vi "AmplitudeModulation.vi"() -> ()   [LabVIEW 2015]
uses:
  <vilib>/DAQmx/read.llb/DAQmx Read (Analog 1D DBL NChan 1Samp).vi
  <vilib>/DAQmx/miscellaneous.llb/DAQmx Fill In Error Info.vi
  <vilib>/addons/control/pid/pid.llb/PID (DBL).vi
  <instrlib>/Agilent 33XXX Series/Agilent 33XXX Series.lvlib
  <vilib>/addons/control/pid/NI_PID_pid.lvlib
  <vilib>/ptbypt/NI_PtbyPt.lvlib
panel:
  in  "View Saved Data\nUpon Completion":bool=TRUE
  out "Time Elapsed (s)":u32
  out "Temperature":dbl[](graph) caption="Signals"
  in  "Slide":dbl(slide) scale=35.0..45.0
  in  "Start":bool
  out "Actual Samp\nRate (Hz)":dbl format="%#_2g"
  in  "Feed back Mechanism":enum32{"PID Control", "Simple P Control"}(tab)
  in  "PID gains":T1={"proportional gain (Kc)"=0.03, "integral time (Ti, min)"=0.175, "derivative time (Td, min)"=0.003} {"derivative time (Td, min)" format="%.3f"; "integral time (Ti, min)" format="%.3f"; "proportional gain (Kc)" format="%.3f"}
  in  "Simple P":dbl
  in  "Amplitude\nModulation?":bool=TRUE
  in  "voltage limit":dbl=0.3 format="%#_13g"
  in  "Set Point (C)":dbl=40.0
  in  "Total Time (s)":u32=300
  in  "Output":bool=TRUE
  in  "Amplitude (V)":dbl=0.2 format="%#_3g"
  in  "Stop":bool
  out "Current Reading":dbl=34.489131869267396 format="%#.1g"
  out "Waveform Chart":waveform(dbl)(graph)
  in  "Log Data?":bool=TRUE
  in  "Description":string="Test Data. See Pictures."
  in  "File Path":path=path "C:/Data/Sonify Labview/ChickenWithChillerWithStandoff.lvm" caption="Filename"
  # "(Set Point - Current Reading) * P\n+ Current Voltage\n= New Voltage"
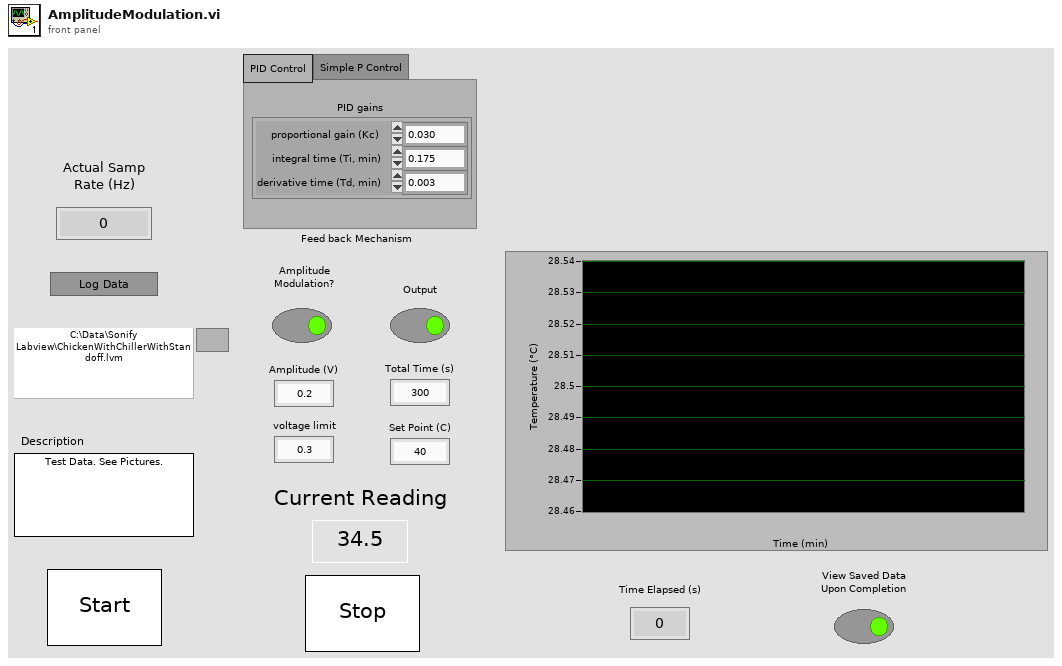
[diagram p1: front panel]
types:
  T1 = cluster{"proportional gain (Kc)":dbl, "integral time (Ti, min)":dbl, "derivative time (Td, min)":dbl}
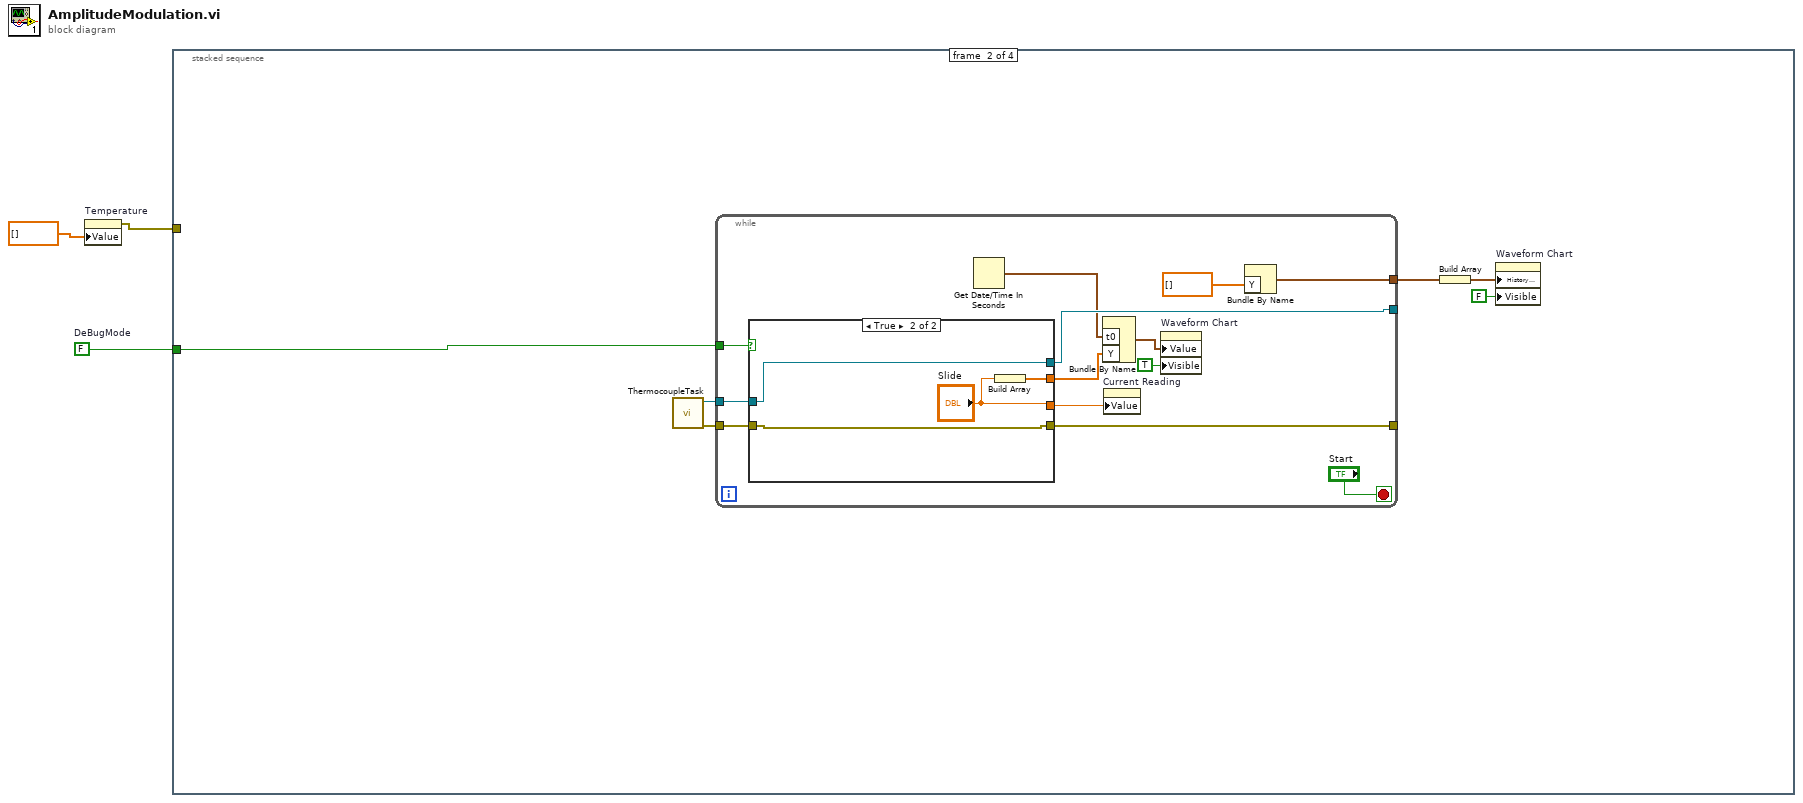
[diagram p0: block diagram]
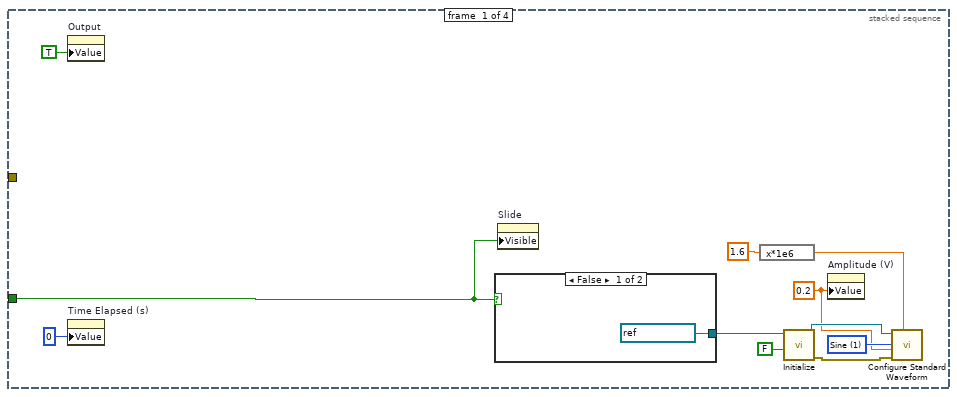
[diagram p2: hidden frame]
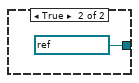
[diagram p3: hidden frame]
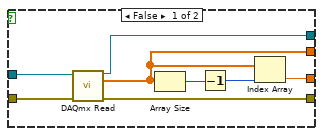
[diagram p4: hidden frame]
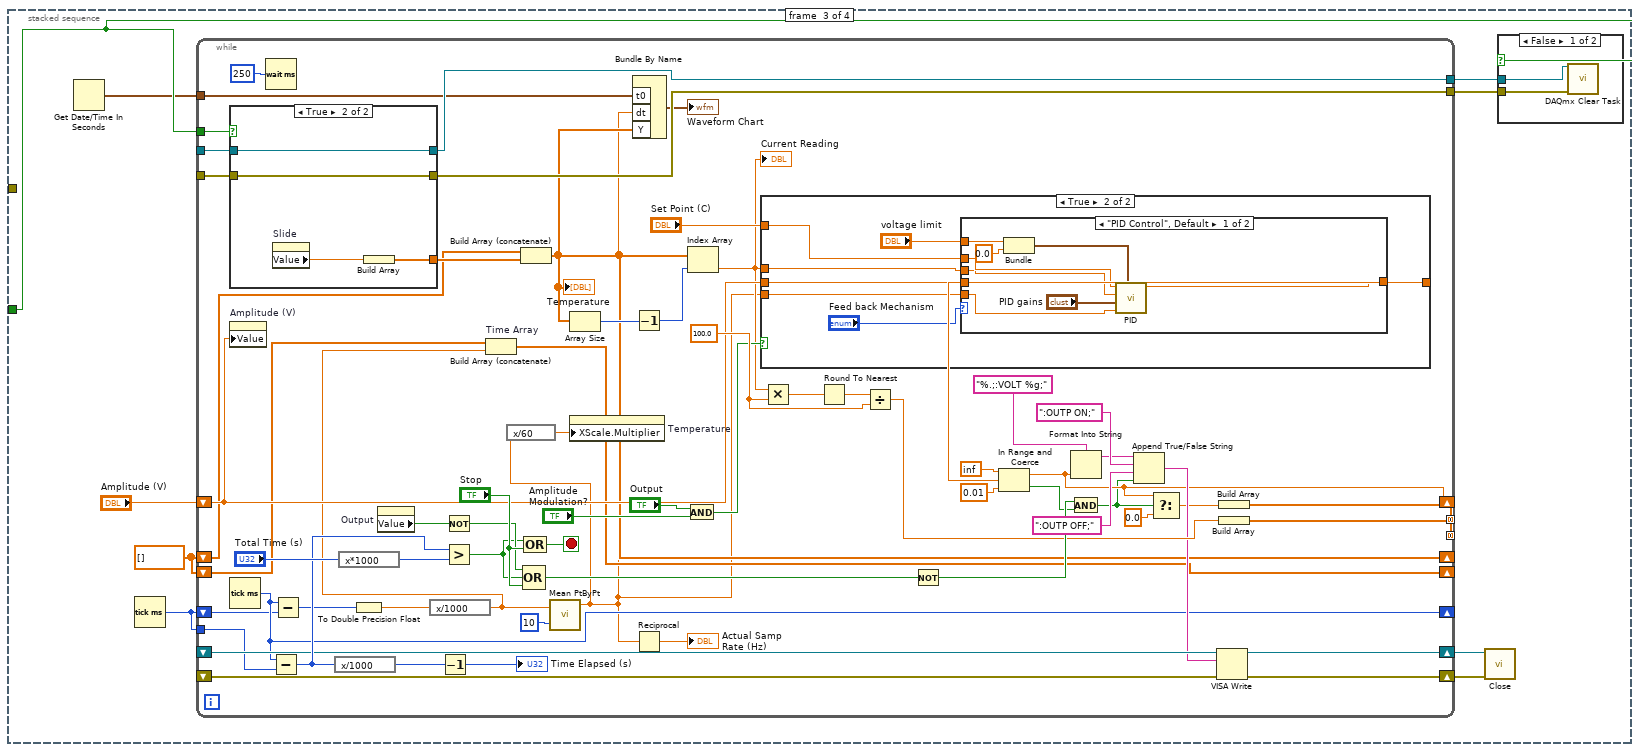
[diagram p5: hidden frame]
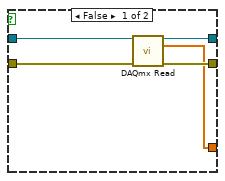
[diagram p7: hidden frame]
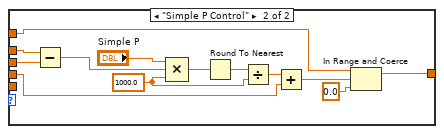
[diagram p9: hidden frame]
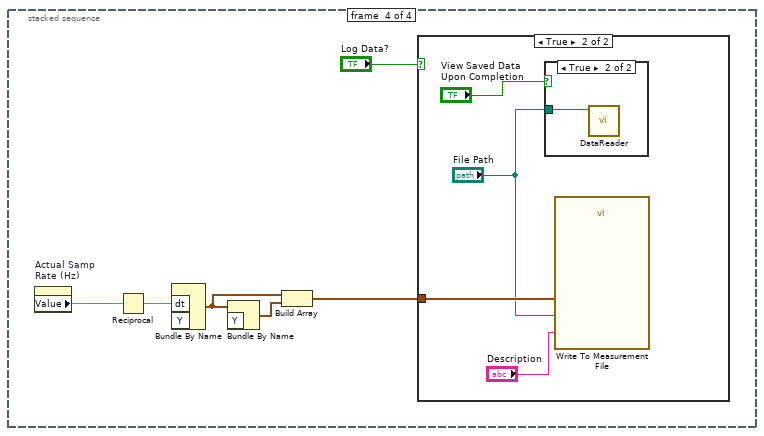
[diagram p10: hidden frame]
diagram:
  w3 = FALSE  # DeBugMode
  n1 = property on="Temperature" class="WFGraph (strict)"("Value"=dbl[] []) -> (error out=w2:errorcluster)  [unwired: 2 in, 1 out]
  n2 = stacked-sequence {
    seq-local: [_ _ w64 _] -> [_ _ _ w179]
    seq-local: [w8 _ _ _] -> [_ _ w60 _]
    seq-local: [w7 _ _ _] -> [_ _ w59 _]
    seq-local: [_ w24 _ _] -> [_ _ w57 _]
    seq-local: [_ w23 _ _] -> [_ _ w53 _]
    seq-local: [_ _ w56 _] -> [_ _ _ w177]
    tunnel: w3 -> [w4 w20 w55 _]
    tunnel: w2 -> [_ _ _ _]
    frame #0 {
      w10 = u16 1 items=["DC", "Sine", "Square", "Triangle", "Ramp", "Pulse", "Noise", "Sinc", "Negative Ramp", "Exponential Rise", "Exponential Fall", "Cardiac"] ("Waveform Function (1: Sine)")
      w5 = 0.2 ("Amplitude (1)")
      n3 = property on="Output" class="Bool (strict)"("Value"=TRUE ("Enable Output  (T: Enable)")) -> ()  [unwired: 2 in, 2 out]
      n4 = property on="Time Elapsed (s)" class="DigNum (strict)"("Value"=u32 0 ("Time Elapsed (s)")) -> ()  [unwired: 2 in, 2 out]
      n5 = case shown="False" w4 {
        tunnel: [refnum<visa-resource-name> "FunGen1" ("Function Gen Address") refnum<visa-resource-name> "FunGen2" ("Function Gen Address")] -> w14
        frame False {
        }
        frame True {
        }
      }
      n6 = property on="Slide" class="Slide (strict)"("Visible"=w4) -> ()  [unwired: 2 in, 2 out]
      n7 = expression code="x*1e6"(1.6 ("Frequency (1000 Hz)")) -> (w6:dbl)
      n8 = call <instrlib>:"Initialize.vi"("Reset (True)"=FALSE, "VISA resource name"=w14) -> ("error out"=w12:errorcluster, "VISA resource name out"=w13:refnum<visa-resource-name>)  [unwired: 8 in]
      n9 = property on="Amplitude (V)" class="DigNum (strict)"("Value"=w5) -> ()  [unwired: 2 in, 2 out]
      n10 = call <instrlib>:"Configure Standard Waveform.vi"("Frequency (1000 Hz)"=w6, "error in (no error)"=w12, "Amplitude (1)"=w5, "Waveform Function (1: Sine)"=w10, "VISA resource name"=w13) -> ("error out"=w7:errorcluster, "VISA resource name out"=w8:refnum<visa-resource-name>)  [unwired: 5 in]
    }
    frame #1 {
      n11 = call "ThermocoupleTask.vi"() -> ("error out"=w25:errorcluster, "task out"=w26:refnum<k21>)  [unwired: 10 in]
      n12 = while {
        tunnel: w26 -> [w39]
        tunnel: w25 -> [w38]
        tunnel: [w34] -> w24
        tunnel: [w33] -> w23
        tunnel: [w31] -> w22
        tunnel: w20 -> [w29]
        stop <- "Start" stop-if-true
        n13 = case shown="True" w29 {
          tunnel: w39 -> [w47 w51]
          tunnel: w38 -> [w46 w50]
          tunnel: [w43 w48] -> w36
          tunnel: [w42 "Slide"] -> w35
          tunnel: [w41 w51] -> w34
          tunnel: [w40 w50] -> w33
          frame False {
            n14 = call-poly <vilib>:"DAQmx Read.vi"("task/channels in"=w47, "error in"=w46) -> ("task out"=w41:refnum<k21>, "data"=w43:dbl[], "error out"=w40:errorcluster)  [unwired: 11 in]
            n15 = Array Size(array=w43) -> (size(s)=w45:i32)
            n16 = Decrement(x=w45) -> (x-1=w44:i32)
            n17 = Index Array(array=w43, index=w44) -> (element=w42:dbl)
          }
          frame True {
            n18 = Build Array("Slide") -> (w48:dbl[])
          }
        }
        n19 = Get Date/Time In Seconds() -> (seconds since 1Jan1904=w28:timestamp)
        n20 = Bundle By Name("t0"=w28, "Y"=w36) -> (w32:waveform(dbl))  [unwired: 1 in]
        n21 = property on="Current Reading" class="DigNum (strict)"("Value"=w35) -> ()  [unwired: 2 in, 2 out]
        n22 = property on="Waveform Chart" class="WFChart (strict)"("Value"=w32, "Visible"=TRUE) -> ()  [unwired: 2 in, 2 out]
        n23 = Bundle By Name("Y"=dbl[] []) -> (w31:waveform(dbl))  [unwired: 1 in]
      }
      n24 = Build Array(w22) -> (w21:waveform(dbl)[])
      n25 = property on="Waveform Chart" class="WFChart (strict)"("History Data"=w21, "Visible"=FALSE) -> ()  [unwired: 2 in, 2 out]
    }
    frame #2 {
      w52 = dbl[] []
      n26 = Get Date/Time In Seconds() -> (seconds since 1Jan1904=w54:timestamp)
      n27 = Tick Count (ms)() -> (millisecond timer value=w61:u32)
      n28 = while {
        shift-right: [w111] -> w66
        shift-left: w59 -> [w109]
        shift-right: [w112] -> w65
        shift-left: w60 -> [w110]
        tunnel: w61 -> [w102]
        shift-right: [w84] -> _
        shift-left: "Amplitude (V)" -> [w108]
        tunnel: [w126] -> w64 mode=concatenating
        shift-right: [w93] -> _
        shift-left: w61 -> [w92]
        tunnel: w57 -> [w98]
        tunnel: [w97] -> w63
        tunnel: [w96] -> w62
        tunnel: w53 -> [w95]
        tunnel: [w80] -> w56 mode=concatenating
        tunnel: w55 -> [w78]
        shift-right: [w75] -> _
        shift-left: w52 -> [w76]
        tunnel: w54 -> [w74]
        shift-right: [w71] -> _
        shift-left: w52 -> [w73]
        stop <- w134 stop-if-true
        w122 = 100.0 ("y")
        n29 = case shown="True" w78 {
          tunnel: w98 -> [w139 w141]
          tunnel: [w138 w141] -> w97
          tunnel: [w137 w140] -> w96
          tunnel: w95 -> [w136 w140]
          tunnel: [w135 w142] -> w77
          frame False {
            n30 = call-poly <vilib>:"DAQmx Read.vi"("task/channels in"=w139, "error in"=w136) -> ("task out"=w138:refnum<k21>, "data"=w135:dbl[], "error out"=w137:errorcluster)  [unwired: 11 in]
          }
          frame True {
            n31 = property on="Slide" class="Slide (strict)"() -> ("Value"=w143:dbl)  [unwired: 2 in, 2 out]
            n32 = Build Array(w143) -> (w142:dbl[])
          }
        }
        n33 = property on="Amplitude (V)" class="DigNum (strict)"("Value"=w108) -> ()  [unwired: 2 in, 2 out]
        n34 = Tick Count (ms)() -> (millisecond timer value=w93:u32)
        n35 = Wait (ms)(milliseconds to wait=u32 250) -> ()  [unwired: 1 out]
        n36 = Subtract(x=w93, y=w102) -> (x-y=w114:u32)
        n37 = Subtract(x=w93, y=w92) -> (x-y=w91:u32)
        n38 = expression code="x/1000"(w114) -> (w87:u32)
        n39 = expression code="x*1000"("Total Time (s)") -> (w132:u32)
        n40 = To Double Precision Float(number=w91) -> (double precision float=w89:dbl)
        n41 = property on="Output" class="Bool (strict)"() -> ("Value"=w128:bool)  [unwired: 2 in, 2 out]
        n42 = expression code="x/1000"(w89) -> (w72:dbl)
        n43 = Decrement(x=w87) -> (x-1=→"Time Elapsed (s)":u32)
        n44 = Not(x=w128) -> (.not. x?=w121:bool)
        n45 = Greater?(x=w114, y=w132) -> (0:w120:bool)
        n46 = Build Array (concatenate) "Time Array"(w73, w72) -> (w71:dbl[])
        n47 = Build Array (concatenate)(w76, w77) -> (w75:dbl[])
        "Temperature" <- w75
        n48 = Compound Arithmetic op=OR(w121, w120, "Stop") -> (w130:bool)
        n49 = Compound Arithmetic op=OR(w120, "Stop") -> (w134:bool)
        n50 = call <vilib>:"Mean PtByPt.vi"("x"=w72, "sample length"=10) -> ("mean"=w70:dbl)  [unwired: 2 in, 1 out]
        n51 = expression code="x/60"(w70) -> (w69:dbl)
        n52 = Array Size(array=w75) -> (size(s)=w100:i32)
        n53 = property on="Temperature" class="WFGraph (strict)"("XScale.Multiplier"=w69) -> ()  [unwired: 2 in, 2 out]
        n54 = Bundle By Name("t0"=w74, "dt"=w70, "Y"=w75) -> (→"Waveform Chart":waveform(dbl))  [unwired: 1 in]
        n55 = Decrement(x=w100) -> (x-1=w99:i32)
        n56 = Reciprocal(x=w70) -> (1/x=→"Actual Samp\nRate (Hz)":dbl)
        n57 = And(x="Output", y="Amplitude\nModulation?") -> (x .and. y?=w115:bool)
        n58 = Index Array(array=w75, index=w99) -> (element=w101:dbl)
        "Current Reading" <- w101
        n59 = case shown="True" w115 {
          tunnel: w101 -> [_ w150]
          tunnel: [w144 w148] -> w113
          tunnel: w108 -> [w144 w149]
          tunnel: "Set Point (C)" -> [_ w151]
          tunnel: w70 -> [_ w146]
          frame False {
          }
          frame True {
            n60 = case shown="\"PID Control\", Default" "Feed back Mechanism" {
              tunnel: w151 -> [w155 w169]
              tunnel: w150 -> [w153 w168]
              tunnel: w149 -> [_ w166]
              tunnel: [w156 w163] -> w148
              tunnel: "voltage limit" -> [w154 w165]
              tunnel: w146 -> [w152 _]
              frame "PID Control", Default {
                n61 = Bundle("voltage limit"=w154, "output low"=0.0) -> (w159:cluster{"voltage limit":dbl, "output low":dbl})  [unwired: 1 in]
                n62 = call-poly <vilib>:"PID.vi"("output range"=w159, "dt (s)"=w152, "PID gains"="PID gains", "process variable"=w153, "setpoint"=w155) -> ("output"=w156:dbl)  [unwired: 5 in, 1 out]
              }
              frame "Simple P Control" {
                w170 = 1000.0 ("y")
                n63 = Subtract(x=w169, y=w168) -> (x-y=w161:dbl)
                n64 = Compound Arithmetic op=MULTIPLY("Simple P", w161, w170) -> (w172:dbl)
                n65 = Round To Nearest(number=w172) -> (nearest integer value=w171:dbl)
                n66 = Divide(x=w171, y=w170) -> (x/y=w167:dbl)
                n67 = Add(x=w167, y=w166) -> (x+y=w164:dbl)
                n68 = In Range and Coerce(upper limit=w165, x=w164, lower limit=0.0) -> (coerced(x)=w163:dbl)  [unwired: 1 out]
              }
            }
          }
        }
        n69 = Multiply(x=w101, y=w122) -> (x*y=w125:dbl)
        n70 = Round To Nearest(number=w125) -> (nearest integer value=w124:dbl)
        n71 = Divide(x=w124, y=w122) -> (x/y=w123:dbl)
        n72 = Not(x=w130) -> (.not. x?=w131:bool)
        n73 = In Range and Coerce(upper limit=inf, x=w113, lower limit=0.01) -> (coerced(x)=w84:dbl, In Range?=w116:bool)
        n74 = Format Into String(format string="%.;:VOLT %g;" ("Amplitude Command"), w84) -> (resulting string=w104:string)  [unwired: 2 in, 1 out]
        n75 = And(x=w131, y=w116) -> (x .and. y?=w82:bool)
        n76 = Append True/False String(1:w82, 2:":OUTP OFF;" ("true string"), 3:":OUTP ON;" ("true string"), 4:w104) -> (0:w103:string)
        n77 = Select(t=w84, s=w82, f=0.0) -> (s? t:f=w81:dbl)
        n78 = VISA Write(VISA resource name=w110, write buffer=w103, error in (no error)=w109) -> (VISA resource name out=w112:refnum<visa-resource-name>, error out=w111:errorcluster)  [unwired: 1 out]
        n79 = Build Array(w81) -> (w80:dbl[])
        n80 = Build Array(w123) -> (w126:dbl[])
      }
      n81 = call <instrlib>:"Close.vi"("error in (no error)"=w66, "VISA resource name"=w65) -> ()  [unwired: 9 in, 1 out]
      n82 = case shown="False" w55 {
        tunnel: w63 -> [w68 _]
        tunnel: w62 -> [w67 _]
        frame False {
          n83 = call <vilib>:"DAQmx Clear Task.vi"("task in"=w68, "error in"=w67) -> ()  [unwired: 13 in, 1 out]
        }
        frame True {
        }
      }
    }
    frame #3 {
      n84 = property on="Actual Samp\nRate (Hz)" class="DigNum (strict)"() -> ("Value"=w178:dbl)  [unwired: 2 in, 2 out]
      n85 = Reciprocal(x=w178) -> (1/x=w173:dbl)
      n86 = Bundle By Name("dt"=w173, "Y"=w179) -> (w174:waveform(dbl))  [unwired: 1 in]
      n87 = Bundle By Name(cluster=w174, "Y"=w177) -> (w176:waveform(dbl))
      n88 = Build Array(w174, w176) -> (w175:waveform(dbl)[])
      n89 = case shown="True" "Log Data?" {
        tunnel: w175 -> [_ w183]
        frame False {
        }
        frame True {
          n90 = case shown="True" "View Saved Data\nUpon Completion" {
            tunnel: "File Path" -> [_ w185]
            frame False {
            }
            frame True {
              n91 = call "DataReader.vi"("Filename"=w185) -> ()  [unwired: 11 in]
            }
          }
          n92 = call "Write To Measurement File"("Signals"=w183, "Filename"="File Path", "Comment"="Description") -> ()  [unwired: 14 in, 3 out]
        }
      }
    }
  }
